vi "Rohde & Schwarz VNA Set Channel.vi"(7 "Rohde & Schwarz VNA":T1, 8 "error in (no error)":errorcluster, 10 "Channel":i8=1 min=1 max=99 step=1, 11 "VISA Resource Name":refnum<visa-resource-name>) -> (0 "error out":errorcluster, 3 "dup VISA Resource Name":refnum<visa-resource-name>)   [LabVIEW 2011]
uses:
  TypeDefs/Rohde & Schwarz VNA Instrument Info.ctl
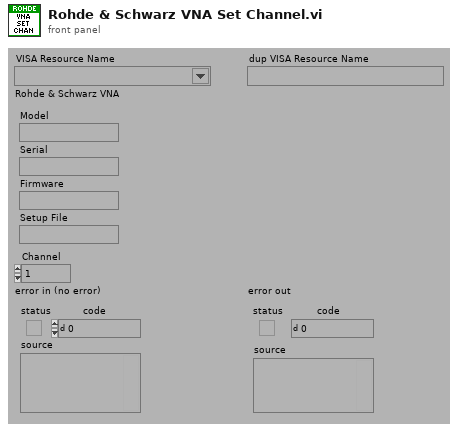
[diagram p1: front panel]
types:
  T1 = typedef "Rohde & Schwarz VNA Instrument Info.ctl" = cluster{"Model":string, "Serial":string, "Firmware":string, "Setup File":string}
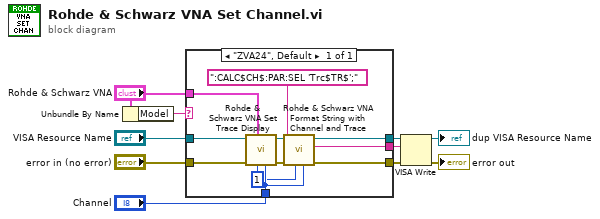
[diagram p0: block diagram]
diagram:
  n1 = Unbundle By Name("Rohde & Schwarz VNA") -> ("Model"=w2:string)
  n2 = case shown="\"ZVA24\", Default" w2 {
    tunnel: "VISA Resource Name" -> [w18]
    tunnel: "error in (no error)" -> [w17]
    tunnel: [w15] -> w6
    tunnel: [w16] -> w5
    tunnel: "Rohde & Schwarz VNA" -> [w19]
    tunnel: "Channel" -> [w12]
    tunnel: [w13] -> w1
    frame "ZVA24", Default {
      w11 = i8 1 ("Channel")
      n3 = call "Rohde & Schwarz VNA Set Trace Display.vi"("Trace"=w12, "Channel"=w11, "Rohde & Schwarz VNA"=w19, "error in (no error)"=w17, "VISA Resource Name"=w18) -> ("error out"=w16:errorcluster, "dup VISA Resource Name"=w15:refnum<visa-resource-name>)  [unwired: 5 out]
      n4 = call "Rohde & Schwarz VNA Format String with Channel and Trace.vi"("Trace"=w12, "Channel"=w11, "String"=":CALC$CH$:PAR:SEL 'Trc$TR$';") -> ("String Out"=w13:string)  [unwired: 6 out]
    }
  }
  n5 = VISA Write(VISA resource name=w6, write buffer=w1, error in (no error)=w5) -> (VISA resource name out=→"dup VISA Resource Name":refnum<visa-resource-name>, error out=→"error out":errorcluster)  [unwired: 1 out]
